vi "BASE.LoadConfig.vi"(8 "error in (no error)":errorcluster, 10 "config file path":path, 11 "BASE in":refnum<class "BASE.lvclass">) -> (0 "error out":errorcluster, 3 "BASE out":refnum<class "BASE.lvclass">)   [LabVIEW 2019, in "BASE.lvlib" / "BASE.lvclass"]
uses:
  BASE.lvclass
  BASE.lvclass/BASE.ctl
  <vilib>/Utility/config.llb/NI_LVConfig.lvlib
panel:
  out "class name":string
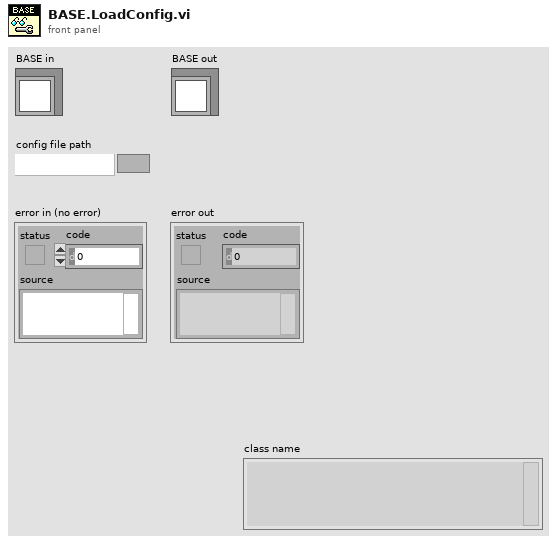
[diagram p1: front panel]
types:
  T1 = typedef "BASE.lvlib/BASE.lvclass/config--cluster.ctl" = cluster{"Path":path}
  T2 = typedef "NI_LVConfig.lvlib/Config Data RefNum.ctl" = refnum<k1>
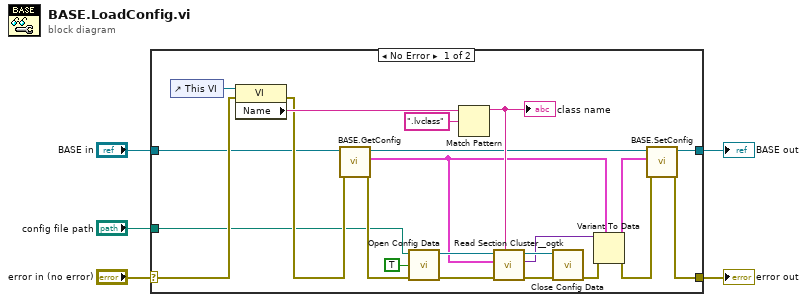
[diagram p0: block diagram]
diagram:
  n1 = case shown="No Error" "error in (no error)" {
    selector: "error in (no error)" -> [w15 w28]
    tunnel: [w7 w28] -> w4
    tunnel: [w10 w27] -> w2
    tunnel: "BASE in" -> [w11 w27]
    tunnel: "config file path" -> [w6 _]
    frame No Error {
      n2 = control-ref of="This VI"() -> (w21:refnum<vi>)
      n3 = property class="VI"(reference=w21, error in=w15) -> (error out=w17:errorcluster, "Name"=w20:string)  [unwired: 1 out]
      n4 = call "BASE.GetConfig.vi"("error in (no error)"=w17, "BASE in"=w11) -> ("error out"=w22:errorcluster, "Config"=w13:T1, "BASE out"=w10:refnum<class "BASE.lvclass">)  [unwired: 7 in]
      n5 = call <vilib>:"Open Config Data.vi"("error in (no error)"=w22, "create file if necessary (T)"=TRUE, "configuration file path"=w6) -> ("error out"=w25:errorcluster, "refnum"=w26:T2)  [unwired: 6 in, 1 out]
      n6 = Match Pattern(string=w20, regular expression=".lvclass") -> (before substring=w18:string)  [unwired: 1 in, 3 out]
      "class name" <- w18
      n7 = call <userlib>:"Read Section Cluster__ogtk.vi"("section (optional)"=w18, "error in (no error)"=w25, "Section Formatted Cluster Type"=w13, "refnum"=w26) -> ("error out"=w24:errorcluster, "Section Formatted Cluster"=w14:variant, "dup refnum"=w23:T2)  [unwired: 3 in, 2 out]
      n8 = call <vilib>:"Close Config Data.vi"("error in (no error)"=w24, "refnum"=w23) -> ("error out"=w9:errorcluster)  [unwired: 8 in, 1 out]
      n9 = Variant To Data(error in=w9, type=w13, Variant=w14) -> (data=w12:T1, error out=w8:errorcluster)
      n10 = call "BASE.SetConfig.vi"("error in (no error)"=w8, "Config"=w12, "BASE in"=w10) -> ("error out"=w7:errorcluster)  [unwired: 7 in, 1 out]
    }
    frame Error {
    }
  }
  "error out" <- w4
  "BASE out" <- w2
